vi "Add Fake Hardware Custom Device.vi"(8 "error in (no error)":errorcluster, 10 "Slot Number":i32, 11 "SLSC Chassis Ref":u64) -> (0 "error out":errorcluster, 2 "Fake Hardware Custom Device Ref":T1 format="%.0x", 3 "SLSC Chassis Ref out":u64)   [LabVIEW 2017, in "Fake Hardware Custom Device.lvlib"]
uses:
  Fake Hardware Custom Device.lvlib
  <vilib>/NI Veristand/Custom Device API/Custom Device Item Ref.ctl
  <userlib>/_OpenG.lib/file/file.llb/Append Path to Root if Relative - Scalar__ogtk.vi
  Shared/VeriStand SLSC Scripting/VeriStand SLSC Scripting.lvlib
  niveristand-custom-device-testing-tools/VeriStandTestUtilities/VeriStandTestUtilities.lvlib
  <vilib>/NI Veristand/Custom Device API/Custom Device API.lvlib
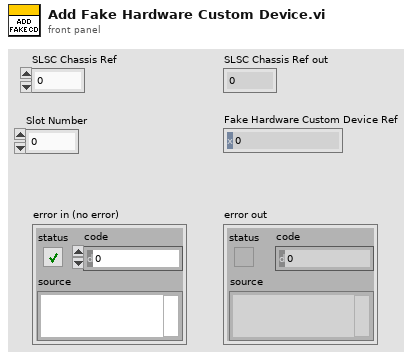
[diagram p1: front panel]
types:
  T1 = typedef "Custom Device API.lvlib/Custom Device Item Ref.ctl" = u64
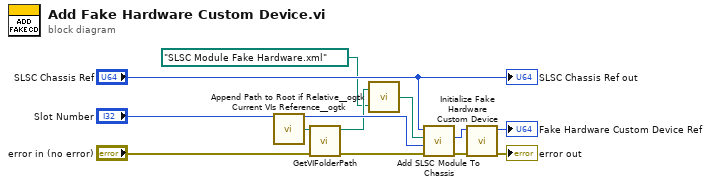
[diagram p0: block diagram]
diagram:
  n1 = call <userlib>:"Current VIs Reference__ogtk.vi"() -> ("Current VI's reference"=w7:refnum<vi>)  [unwired: 5 in]
  n2 = call "GetVIFolderPath.vi"("error in (no error)"="error in (no error)", "VI Reference in"=w7) -> ("error out"=w4:errorcluster, "VI Folder Path out"=w6:path)  [unwired: 8 in]
  n3 = call-poly <userlib>:"Append Path to Root if Relative__ogtk.vi"("Absolute or Relative Path"=path "SLSC Module Fake Hardware.xml", "Root Path"=w6) -> ("Absolute or Appended Path"=w3:path)
  n4 = call "Add SLSC Module To Chassis.vi"("error in (no error)"=w4, "Slot Number"="Slot Number", "SLSC Custom Device XML"=w3, "SLSC Chassis"="SLSC Chassis Ref") -> ("error out"=w12:errorcluster, "SLSC Module"=w11:u64)  [unwired: 5 in, 1 out]
  n5 = call "Initialize Fake Hardware Custom Device.vi"("error in (no error)"=w12, "Hardware Ref in"=w11) -> ("error out"=→"error out":errorcluster, "Hardware Ref out"=→"Fake Hardware Custom Device Ref":T1)  [unwired: 8 in]
  "SLSC Chassis Ref out" <- "SLSC Chassis Ref"
